vi "test22-TestArgumentInfoOfTriggeredState_State.vi"(8 "error in (no error)":errorcluster, 11 "TestCase in":refnum<class "testcase-CSMBroadcast.lvclass">) -> (0 "error out":errorcluster, 3 "TestCase out":refnum<class "testcase-CSMBroadcast.lvclass">)   [LabVIEW 2017, in "testcase-CSMBroadcast.lvclass"]
uses:
  testcase-CSMBroadcast.lvclass
  bc269a46-fbd8-4fbd-ac76-06990d02385a.vi
  8d37a2f4-20d8-4102-818c-5a8acec6f80e.vi
  src/user.lib/_NEVSTOP/Communicable State Machine(CSM)/AdvanceAPI/CSM - Get Module Attribute.vi
  <vilib>/addons/_JKI Toolkits/VI Tester/TestCase.llb/TestCase.lvclass
  src/user.lib/_NEVSTOP/Communicable State Machine(CSM)/Communicable State Machine.lvlib
  CSM/CSM-Testcase.lvlib
  C:/Program Files (x86)/National Instruments/LabVIEW 2017/vi.lib/addons/_JKI Toolkits/VI Tester/TestCase.llb/TestCase.lvclass
panel:
  out "LoopCount":i32
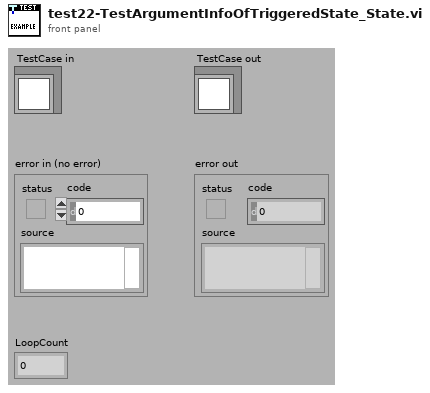
[diagram p1: front panel]
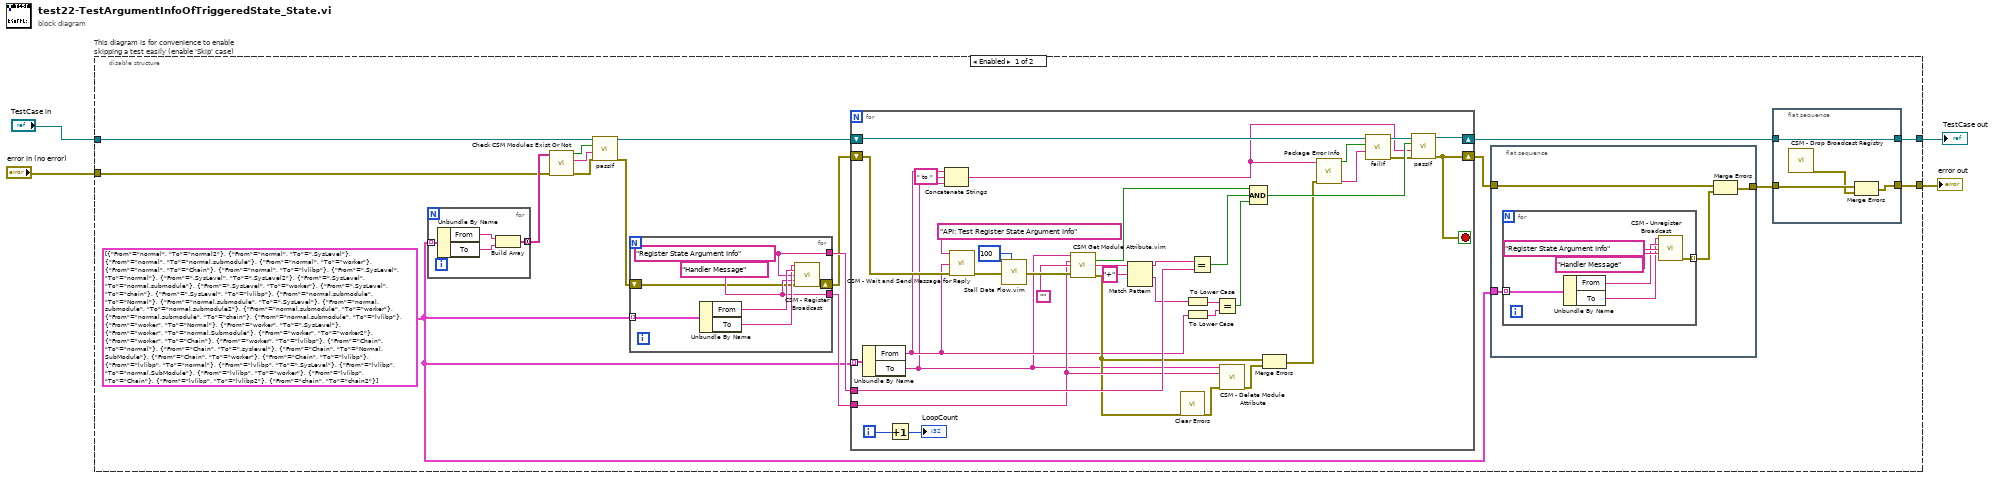
[diagram p0: block diagram]
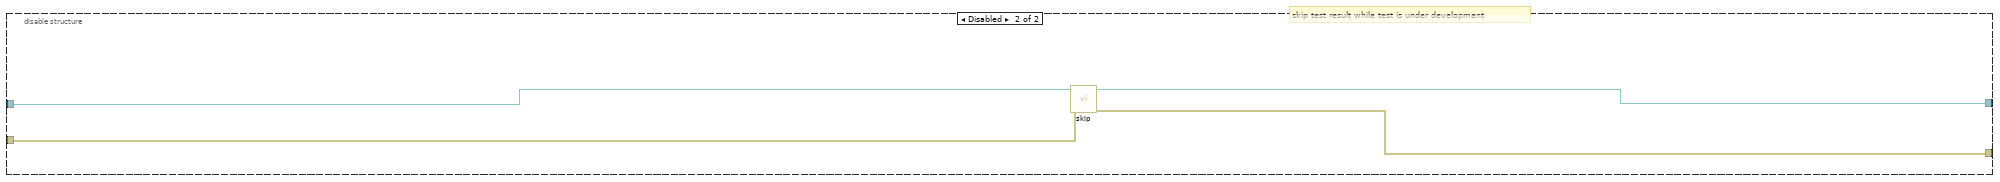
[diagram p2: hidden frame]
diagram:
  n1 = disable-structure "This diagram is for convenience to enable skipping a test easily (enable 'Skip' case)" shown="Enabled" {
    disable-tunnel: "TestCase in" -> [w9 w86]
    disable-tunnel: [w16 w84] -> w2
    disable-tunnel: [w19 w85] -> w1
    disable-tunnel: "error in (no error)" -> [w8 w83]
    frame Enabled {
      w10 = cluster{"From":string, "To":string}[] [{"From"="normal", "To"="normal2"}, {"From"="normal", "To"=".SysLevel"}, {"From"="normal", "To"="normal.submodule"}, {"From"="normal", "To"="worker"}, {"From"="normal", "To"="Chain"}, {"From"="normal", "To"="lvlibp"}, {"From"=".SysLevel", "To"="normal"}, {"From"=".SysLevel", "To"=".SysLevel2"}, {"From"=".SysLevel", "To"="normal.submodule"}, {"From"=".SysLevel", "To"="worker"}, {"From"=".SysLevel", "To"="chain"}, {"From"=".SysLevel", "To"="lvlibp"}, {"From"="normal.submodule", "To"="Normal"}, {"From"="normal.submodule", "To"=".SysLevel"}, {"From"="normal.submodule", "To"="normal.submodule2"}, {"From"="normal.submodule", "To"="worker"}, {"From"="normal.submodule", "To"="chain"}, {"From"="normal.submodule", "To"="lvlibp"}, {"From"="worker", "To"="Normal"}, {"From"="worker", "To"=".SysLevel"}, {"From"="worker", "To"="normal.Submodule"}, {"From"="worker", "To"="worker2"}, {"From"="worker", "To"="Chain"}, {"From"="worker", "To"="lvlibp"}, {"From"="Chain", "To"="normal"}, {"From"="Chain", "To"=".syslevel"}, {"From"="Chain", "To"="Normal.SubModule"}, {"From"="Chain", "To"="worker"}, {"From"="Chain", "To"="lvlibp"}, {"From"="lvlibp", "To"="normal"}, {"From"="lvlibp", "To"=".SysLevel"}, {"From"="lvlibp", "To"="normal.SubModule"}, {"From"="lvlibp", "To"="worker"}, {"From"="lvlibp", "To"="Chain"}, {"From"="lvlibp", "To"="lvlibp2"}, {"From"="chain", "To"="chain2"}]
      n2 = for {
        tunnel: w10 -> [w25] mode=indexing
        tunnel: [w22] -> w13 mode=concatenating
        n3 = Unbundle By Name(w25) -> ("From"=w24:string, "To"=w23:string)
        n4 = Build Array(w24, w23) -> (w22:string[])
      }
      n5 = call "Check CSM Modules Exist Or Not.vi"("error in"=w8, "CSM names in"=w13) -> ("error out"=w11:errorcluster, "Debug string"=w12:string, "All Modules Exist?"=w14:bool)  [unwired: 7 in]
      n6 = call-dynamic "passIf.vi"("error in (no error)"=w11, "message (\"\")"=w12, "pass"=w14, "TestCase in"=w9) -> ("error out"=w6:errorcluster, "TestCase out"=w7:refnum<class "testcase-CSMBroadcast.lvclass">)  [unwired: 6 in]
      n7 = for {
        tunnel: w10 -> [w42] mode=indexing
        tunnel: [w38] -> w18
        tunnel: [w37] -> w15
        shift-right: [w39] -> w5
        shift-left: w6 -> [w36]
        w37 = "Handler Message" ("Response Message (If \"\", Same as Source Message)")
        w38 = "Register State Argument Info" ("Status")
        n8 = Unbundle By Name(w42) -> ("From"=w41:string, "To"=w40:string)
        n9 = call "CSM - Register Broadcast.vi"("CSM Name(Empty for Broadcast Event)"=w40, "Source CSM Name (* as Default)"=w41, "Trigger"=w38, "API (If \"\", Same as Trigger)"=w37, "Error In"=w36) -> ("error out"=w39:errorcluster)  [unwired: 9 in, 1 out]
      }
      n10 = for {
        tunnel: w10 -> [w81] mode=indexing
        shift-right: [w66] -> w17
        shift-left: w7 -> [w57]
        shift-right: [w64] -> w21
        shift-left: w5 -> [w54]
        tunnel: w18 -> [w72]
        tunnel: w15 -> [w63]
        i -> [w61]
        stop <- w64 stop-if-true
        n11 = Unbundle By Name(w81) -> ("From"=w50:string, "To"=w49:string)
        n12 = Increment(x=w61) -> (x+1=→"LoopCount":i32)
        n13 = Concatenate Strings(w50, " to " ("string"), w49) -> (w47:string)
        n14 = call "CSM - Wait and Send Message for Reply.vi"("State"="API: Test Register State Argument Info", "Target Module"=w50, "Error In (No Error)"=w54) -> ("error out"=w80:errorcluster)  [unwired: 9 in, 3 out]
        n15 = call "Stall Data Flow.vim"("value in"=w80, "milliseconds to wait"=u32 100) -> ("value out"=w78:errorcluster)  [unwired: 1 out]
        n16 = call "CSM Get Module Attribute.vim"("CSM Name"=w49, "Attribute"=w63, "Default Value (Empty Variant)"="", "Error In"=w78) -> ("Found"=w76:bool, "Value"=w75:string, "error out"=w53:errorcluster)  [unwired: 7 in, 2 out]
        n17 = Match Pattern(string=w75, regular expression="+") -> (before substring=w73:string, after substring=w71:string)  [unwired: 1 in, 2 out]
        n18 = call <vilib>:"Clear Errors.vi"("error in (no error)"=w53) -> ("error out"=w62:errorcluster)  [unwired: 5 in, 1 out]
        n19 = To Lower Case(string=w50) -> (all lower case string=w69:string)
        n20 = To Lower Case(string=w71) -> (all lower case string=w70:string)
        n21 = Equal?(x=w73, y=w72) -> (x = y?=w68:bool)
        n22 = Equal?(x=w70, y=w69) -> (x = y?=w67:bool)
        n23 = call "CSM - Delete Module Attribute.vi"("CSM Name"=w49, "Attribute"=w63, "Error In"=w62) -> ("error out"=w52:errorcluster)  [unwired: 9 in, 3 out]
        n24 = Compound Arithmetic op=AND(w76, w68, w67) -> (w65:bool)
        n25 = Merge Errors(w53, w52) -> (w51:errorcluster)
        n26 = call "Package Error Info.vi"("error in"=w51, "String in"=w47) -> ("packed error info out"=w58:string, "error status"=w59:bool)  [unwired: 8 in]
        n27 = call-dynamic "failIf.vi"("message (\"\")"=w58, "fail"=w59, "TestCase in"=w57) -> ("error out"=w55:errorcluster, "TestCase out"=w56:refnum<class "testcase-CSMBroadcast.lvclass">)  [unwired: 7 in]
        n28 = call-dynamic "passIf.vi"("error in (no error)"=w55, "message (\"\")"=w47, "pass"=w65, "TestCase in"=w56) -> ("error out"=w64:errorcluster, "TestCase out"=w66:refnum<class "testcase-CSMBroadcast.lvclass">)  [unwired: 6 in]
      }
      n29 = flat-sequence {
        tunnel: w10 -> [w26]
        tunnel: w21 -> [w29]
        tunnel: [w28] -> w20
        frame #0 {
          n30 = for {
            tunnel: w26 -> [w30] mode=indexing
            tunnel: [w31] -> w27 mode=indexing
            n31 = Unbundle By Name(w30) -> ("From"=w33:string, "To"=w32:string)
            n32 = call "CSM - Unregister Broadcast.vi"("CSM Name(Empty for Broadcast Event)"=w32, "Source CSM Name (* as Default)"=w33, "Trigger"="Register State Argument Info" ("Status"), "API (\"*\" as Default)"="Handler Message" ("Response Message (If \"\", Same as Source Message)")) -> ("error out"=w31:errorcluster)  [unwired: 10 in, 1 out]
          }
          n33 = Merge Errors(w29, w27) -> (w28:errorcluster)
        }
      }
      n34 = flat-sequence {
        tunnel: w20 -> [w46]
        tunnel: [w45] -> w19
        tunnel: [w44] -> w16
        tunnel: w17 -> [w44]
        frame #0 {
          n35 = call "CSM - Drop Broadcast Registry.vi"() -> ("error out"=w43:errorcluster)  [unwired: 15 in]
          n36 = Merge Errors(w46, w43) -> (w45:errorcluster)
        }
      }
    }
    frame Disabled {
      # "skip test result while test is under development"
      n37 = call <vilib>:"skip.vi"("error in (no error)"=w83, "TestCase in"=w86) -> ("error out"=w85:errorcluster, "TestCase out"=w84:refnum<class "testcase-CSMBroadcast.lvclass">)  [unwired: 8 in]
    }
  }
  "error out" <- w1
  "TestCase out" <- w2
